vi "Preset Then.vi"(8 "error in (no error)":errorcluster) -> (0 "error out":errorcluster)   [LabVIEW 2017, in "Unit Tests.lvlib"]
uses:
  Unit Tests.lvlib
  Promise Future/Future/Future.lvclass/Future.ctl
  95dc31ad-9ffa-4fc7-be26-3e0641f1d074.vi
  3ca253fc-3f3c-47f3-9a24-db5028bdb027.vi
  b2e5f197-10a3-4ad7-b26c-b44c03cc53a7.vi
  Promise Future/Future/Then.vi
  Promise Future/Promise/Promise.lvclass
  E:/Promise/Promise Future/Future/Future.lvclass
  Basic Then Callback.vi
  Promise Future/Future/Fulfull (Value).vi
  Promise Future/Promise/Read Future.vi
  Promise Future/Future/VI Name Wrapper.vi
  Promise Future/State/Then.vi
  Promise Future/Future/Read Value (private).vi
  Promise Future/Future/Future.lvclass
  <vilib>/addons/_JKI Toolkits/Caraya/classes/Test/Test.lvclass
  <vilib>/addons/_JKI Toolkits/Caraya/classes/Assert/Assert.lvclass
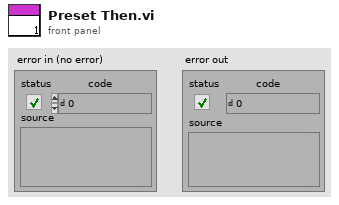
[diagram p1: front panel]
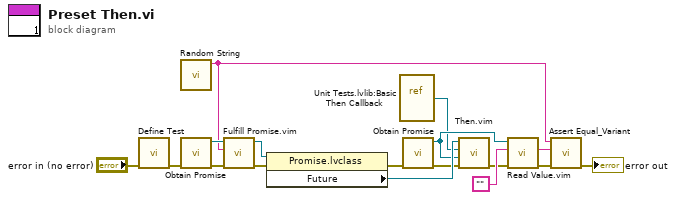
[diagram p0: block diagram]
diagram:
  n1 = call <vilib>:"Define Test.vi"("error in (no error)"="error in (no error)") -> ("error out"=w7:errorcluster)  [unwired: 10 in]
  n2 = call "Random String.vi"() -> ("string"=w2:string)  [unwired: 11 in]
  n3 = call "Obtain Promise.vi"("error in (no error)"=w7) -> ("error out"=w8:errorcluster, "Promise out"=w17:refnum<class "Promise.lvclass">)  [unwired: 8 in, 1 out]
  n4 = call "Fulfill Promise.vim"("error in (no error)"=w8, "Value"=w2, "Promise in"=w17) -> ("error out"=w9:errorcluster, "Promise out"=w5:refnum<class "Promise.lvclass">)  [unwired: 7 in]
  n5 = property class="Promise.lvclass"(reference=w5, error in=w9) -> (error out=w10:errorcluster, "Future"=w16:refnum<class "Future.lvclass">)  [unwired: 1 out]
  n6 = vi-ref "Unit Tests.lvlib:Basic Then Callback.vi"() -> (w1:refnum<vi>)
  n7 = call "Obtain Promise.vi"("error in (no error)"=w10) -> ("error out"=w11:errorcluster, "Promise out"=w4:refnum<class "Promise.lvclass">)  [unwired: 8 in, 1 out]
  n8 = call "Then.vim"("error in (no error)"=w11, "Scope"=w4, "Callback"=w1, "Future in"=w16) -> ("error out"=w12:errorcluster)  [unwired: 6 in, 1 out]
  n9 = call "Read Value.vim"("error in (no error)"=w12, "Default Value"="", "Future in"=w4) -> ("error out"=w14:errorcluster, "Value"=w3:string)  [unwired: 5 in, 2 out]
  n10 = call <vilib>:"Assert Equal_Variant.vi"("error in (no error)"=w14, "Y"=w3, "X"=w2) -> ("error out"=→"error out":errorcluster)  [unwired: 8 in]
